vi "Save Chunk.vi"(8 "error in (no error)":errorcluster, 9 "Volatge":cdb[](array[numeric]), 10 "Frequency":dbl[](array[numeric]), 11 "Spectrum Recorder in":refnum<class "Spectrum Recorder.lvclass">) -> (0 "error out":errorcluster, 3 "Spectrum Recorder out":refnum<class "Spectrum Recorder.lvclass">)   [LabVIEW 2016, in "Spectrum Recorder.lvclass"]
uses:
  Spectrum Recorder.lvclass
  Spectrum Recorder.lvclass/Spectrum Recorder.ctl
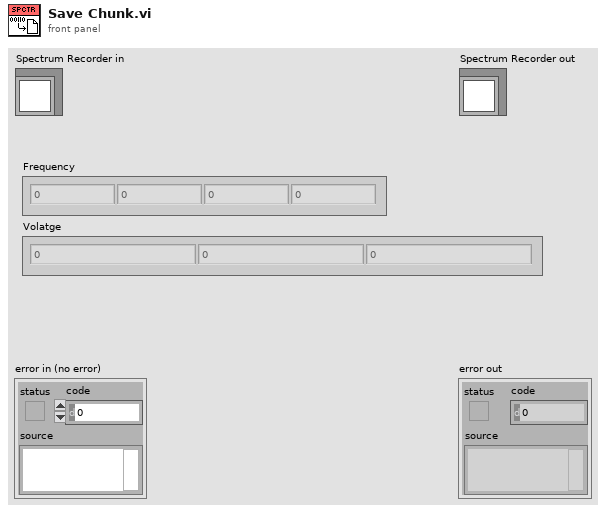
[diagram p1: front panel]
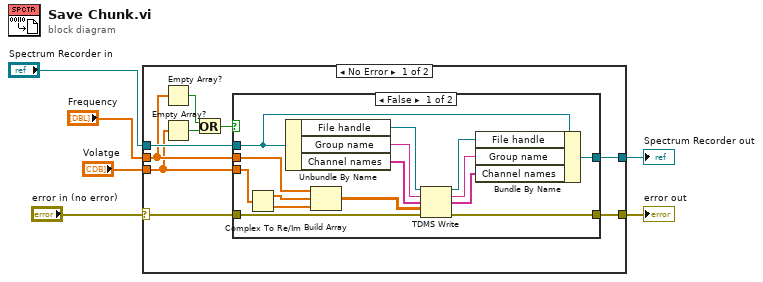
[diagram p0: block diagram]
diagram:
  n1 = case shown="No Error" "error in (no error)" {
    selector: "error in (no error)" -> [w13 w34]
    tunnel: [w12 w34] -> w5
    tunnel: [w14 w33] -> w3
    tunnel: "Spectrum Recorder in" -> [w15 w33]
    tunnel: "Volatge" -> [w7 _]
    tunnel: "Frequency" -> [w8 _]
    frame No Error {
      n2 = Empty Array?(array=w8) -> (empty?=w11:bool)
      n3 = Empty Array?(array=w7) -> (empty?=w10:bool)
      n4 = Or(x=w11, y=w10) -> (x .or. y?=w9:bool)
      n5 = case shown="False" w9 {
        tunnel: w7 -> [w29 _]
        tunnel: w8 -> [w26 _]
        tunnel: w15 -> [w22 w32]
        tunnel: [w18 w32] -> w14
        tunnel: w13 -> [w17 w31]
        tunnel: [w16 w31] -> w12
        frame False {
          n6 = Complex To Re/Im(x + iy=w29) -> (x=w27:dbl[], y=w28:dbl[])
          n7 = Unbundle By Name(w22) -> ("File handle"=w30:refnum<k34>, "Group name"=w24:string, "Channel names"=w23:string[])
          n8 = Build Array(w26, w27, w28) -> (w25:dbl[][])
          n9 = TDMS Write(0:w30, 5:w24, 7:w23, 9:w25, 11:w17) -> (4:w21:refnum<k34>, 6:w20:string, 8:w19:string[], 15:w16:errorcluster)  [unwired: 1 in]
          n10 = Bundle By Name(cluster=w22, "File handle"=w21, "Group name"=w20, "Channel names"=w19) -> (w18:refnum<class "Spectrum Recorder.lvclass">)
        }
        frame True {
        }
      }
    }
    frame Error {
    }
  }
  "error out" <- w5
  "Spectrum Recorder out" <- w3
